vi "ALARM HIGH THRESHOLD 2.vi"(4 "State":i16=-1, 5 "Time":dbl format="%.2f", 6 "Sensor Values":dbl[](array[numeric]), 7 "Set Points":dbl[](array[numeric])=[0.0]) -> (0 "required data":T3={"Set Point names"=["Device ID"], "required number of setpoints"=1, "required number of sensors"=0, "Sensor names"=[]}, 3 "output value":dbl)   [LabVIEW 2019]
uses:
  modbusrtu/MB ID-Address.ctl
  modbusrtu/SerialParameters.ctl
  modbusrtu/MB cmd buffer.ctl
panel:
  in  "ChemTracChannels":string[](array[string])=["Acquiring", "Reserved 1", "Reserved 2", "Reserved 3", "LVAL", "CVAL", "Count Index", "Holding", "Particle Count 1 (high)", "Particle Count 1 (low)", "Particle Count 2 (high)", "Particle Count 2 (low)", "Particle Count 3 (high)", "Particle Count 3 (low)", "Particle Count 4 (high)", "Particle Count 4 (low)", "Particle Count 5 (high)", "Particle Count 5 (low)", "Particle Count 6 (high)", "Particle Count 6 (low)", "Particle Count 7 (high)", "Particle Count 7 (low)", "Particle Count 8 (high)", "Particle Count 8 (low)", "Particle Count 9 (high)", "Particle Count 9 (low)", "Total Counts (high)", "Total Counts (low)", "Alarm Output (0)", "Alarm Output (1)", "Unit Address", "Flow Rate", "Size Ranges 1 (from)", "Size Ranges 1 (to)", "Size Ranges 2 (from)", "Size Ranges 2 (to)", "Size Ranges 3 (from)", "Size Ranges 3 (to)", "Size Ranges 4 (from)", "Size Ranges 4 (to)", "Size Ranges 5 (from)", "Size Ranges 5 (to)", "Size Ranges 6 (from)", "Size Ranges 6 (to)", "Size Ranges 7 (from)", "Size Ranges 7 (to)", "Size Ranges 8 (from)", "Size Ranges 8 (to)", "Sample Frequency", "Sample Time", "CLOCK (year)", "CLOCK (month)", "CLOCK (day)", "CLOCK (hour)", "CLOCK (minute)", "CLOCK (second)", "ALARM HIGH THRESHOLD 1", "ALARM LOW THRESHOLD 1", "ALARM HIGH THRESHOLD 2", "ALARM LOW THRESHOLD 2", "ANALOG INPUT 1-1", "ANALOG INPUT 1-2", "ANALOG INPUT 1-3", "ANALOG INPUT 1-4", "ANALOG INPUT 2-1", "ANALOG INPUT 2-2", "ANALOG INPUT 2-3", "ANALOG INPUT 2-4"]
  in  "MB ID-Address in":T1={"Serial Parameter"={"Mode"=enum."RTU", "Address"=0, "Address bytes"=enum."2 bytes"}, "Start register"=0}
  # "Input Registers (Read Only)\nModbus Map: ChemTrac PC3400 Particle Counter\nAddress\tSize\tType\tDescription\t\t\t\t\t\t\t\t\t\t\t\t\t\n0\t2\tINTEGER\tAcquiring\t\t\t\t\t\t\t\t\t\t\t\t\t\n2\t2\tINTEGER\tReserved 1\t\t\t\t\t\t\t\t\t\t\t\t\t\n4\t2\tINTEGER\tReserved 2\t\t\t\t\t\t\t\t\t\t\t\t\t\n6\t2\tINTEGER\tReserved 3\t\t\t\t\t\t\t\t\t\t\t\t\t\n8\t2\tINTEGER\tLVAL\t\t\t\t\t\t\t\t\t\t\t\t\t\n10\t2\tINTEGER\tCVAL\t\t\t\t\t\t\t\t\t\t\t\t\t\n12\t2\tINTEGER\tCount Index\t\t\t\t\t\t\t\t\t\t\t\t\t\n14\t2\tINTEGER\tHolding\t\t\t\t\t\t\t\t\t\t\t\t\t\n16\t2\tINTEGER\tParticle Count 1 (high)\t\t\t\t\t\t\t\t\t\t\t\t\t\n18\t2\tINTEGER\tParticle Count 1 (low)\t\t\t\t\t\t\t\t\t\t\t\t\t\n20\t2\tINTEGER\tParticle Count 2 (high)\t\t\t\t\t\t\t\t\t\t\t\t\t\n22\t2\tINTEGER\tParticle Count 2 (low)\t\t\t\t\t\t\t\t\t\t\t\t\t\n24\t2\tINTEGER\tParticle Count 3 (high)\t\t\t\t\t\t\t\t\t\t\t\t\t\n26\t2\tINTEGER\tParticle Count 3 (low)\t\t\t\t\t\t\t\t\t\t\t\t\t\n28\t2\tINTEGER\tParticle Count 4 (high)\t\t\t\t\t\t\t\t\t\t\t\t\t\n30\t2\tINTEGER\tParticle Count 4 (low)\t\t\t\t\t\t\t\t\t\t\t\t\t\n32\t2\tINTEGER\tParticle Count 5 (high)\t\t\t\t\t\t\t\t\t\t\t\t\t\n34\t2\tINTEGER\tParticle Count 5 (low)\t\t\t\t\t\t\t\t\t\t\t\t\t\n36\t2\tINTEGER\tParticle Count 6 (high)\t\t\t\t\t\t\t\t\t\t\t\t\t\n38\t2\tINTEGER\tParticle Count 6 (low)\t\t\t\t\t\t\t\t\t\t\t\t\t\n40\t2\tINTEGER\tParticle Count 7 (high)\t\t\t\t\t\t\t\t\t\t\t\t\t\n42\t2\tINTEGER\tParticle Count 7 (low)\t\t\t\t\t\t\t\t\t\t\t\t\t\n44\t2\tINTEGER\tParticle Count 8 (high)\t\t\t\t\t\t\t\t\t\t\t\t\t\n46\t2\tINTEGER\tParticle Count 8 (low)\t\t\t\t\t\t\t\t\t\t\t\t\t\n48\t2\tINTEGER\tParticle Count 9 (high)\t\t\t\t\t\t\t\t\t\t\t\t\t\n50\t2\tINTEGER\tParticle Count 9 (low)\t\t\t\t\t\t\t\t\t\t\t\t\t\n52\t2\tINTEGER\tTotal Counts (high)\t\t\t\t\t\t\t\t\t\t\t\t\t\n54\t2\tINTEGER\tTotal Counts (low)\t\t\t\t\t\t\t\t\t\t\t\t\t\n56\t2\tINTEGER\tAlarm Output (0)\t\t\t\t\t\t\t\t\t\t\t\t\t\n58\t2\tINTEGER\tAlarm Output (1)\t\t\t\t\t\t\t\t\t\t\t\t\t\n60\t1\tINTEGER\tUnit Address\t\t\t\t\t\t\t\t\t\t\t\t\t\n62\t1\tINTEGER\tFlow Rate\t\t\t\t\t\t\t\t\t\t\t\t\t\n64\t2\tINTEGER\tSize Ranges 1 (from)\t\t\t\t\t\t\t\t\t\t\t\t\t\n66\t2\tINTEGER\tSize Ranges 1 (to)\t\t\t\t\t\t\t\t\t\t\t\t\t\n68\t2\tINTEGER\tSize Ranges 2 (from)\t\t\t\t\t\t\t\t\t\t\t\t\t\n70\t2\tINTEGER\tSize Ranges 2 (to)\t\t\t\t\t\t\t\t\t\t\t\t\t\n72\t2\tINTEGER\tSize Ranges 3 (from)\t\t\t\t\t\t\t\t\t\t\t\t\t\n74\t2\tINTEGER\tSize Ranges 3 (to)\t\t\t\t\t\t\t\t\t\t\t\t\t\n76\t2\tINTEGER\tSize Ranges 4 (from)\t\t\t\t\t\t\t\t\t\t\t\t\t\n78\t2\tINTEGER\tSize Ranges 4 (to)\t\t\t\t\t\t\t\t\t\t\t\t\t\n80\t2\tINTEGER\tSize Ranges 5 (from)\t\t\t\t\t\t\t\t\t\t\t\t\t\n82\t2\tINTEGER\tSize Ranges 5 (to)\t\t\t\t\t\t\t\t\t\t\t\t\t\n84\t2\tINTEGER\tSize Ranges 6 (from)\t\t\t\t\t\t\t\t\t\t\t\t\t\n86\t2\tINTEGER\tSize Ranges 6 (to)\t\t\t\t\t\t\t\t\t\t\t\t\t\n88\t2\tINTEGER\tSize Ranges 7 (from)\t\t\t\t\t\t\t\t\t\t\t\t\t\n90\t2\tINTEGER\tSize Ranges 7 (to)\t\t\t\t\t\t\t\t\t\t\t\t\t\n92\t2\tINTEGER\tSize Ranges 8 (from)\t\t\t\t\t\t\t\t\t\t\t\t\t\n94\t2\tINTEGER\tSize Ranges 8 (to)\t\t\t\t\t\t\t\t\t\t\t\t\t\n96\t2\tINTEGER\tSample Frequency\t\t\t\t\t\t\t\t\t\t\t\t\t\n98\t2\tINTEGER\tSample Time\t\t\t\t\t\t\t\t\t\t\t\t\t\n100\t2\tINTEGER\tCLOCK (year)\t\t\t\t\t\t\t\t\t\t\t\t\t\n102\t2\tINTEGER\tCLOCK (month)\t\t\t\t\t\t\t\t\t\t\t\t\t\n104\t2\tINTEGER\tCLOCK (day)\t\t\t\t\t\t\t\t\t\t\t\t\t\n106\t2\tINTEGER\tCLOCK (hour)\t\t\t\t\t\t\t\t\t\t\t\t\t\n108\t2\tINTEGER\tCLOCK (minute)\t\t\t\t\t\t\t\t\t\t\t\t\t\n110\t2\tINTEGER\tCLOCK (second)\t\t\t\t\t\t\t\t\t\t\t\t\t\n112\t2\tINTEGER\tALARM HIGH THRESHOLD 1\t\t\t\t\t\t\t\t\t\t\t\t\t\n114\t2\tINTEGER\tALARM LOW THRESHOLD 1\t\t\t\t\t\t\t\t\t\t\t\t\t\n116\t2\tINTEGER\tALARM HIGH THRESHOLD 2\t\t\t\t\t\t\t\t\t\t\t\t\t\n118\t2\tINTEGER\tALARM LOW THRESHOLD 2\t\t\t\t\t\t\t\t\t\t\t\t\t\n120\t2\tINTEGER\tANALOG INPUT 1-1\t\t\t\t\t\t\t\t\t\t\t\t\t\n122\t2\tINTEGER\tANALOG INPUT 1-2\t\t\t\t\t\t\t\t\t\t\t\t\t\n124\t2\tINTEGER\tANALOG INPUT 1-3\t\t\t\t\t\t\t\t\t\t\t\t\t\n126\t2\tINTEGER\tANALOG INPUT 1-4\t\t\t\t\t\t\t\t\t\t\t\t\t\n128\t2\tINTEGER\tANALOG INPUT 2-1\t\t\t\t\t\t\t\t\t\t\t\t\t\n130\t2\tINTEGER\tANALOG INPUT 2-2\t\t\t\t\t\t\t\t\t\t\t\t\t\n132\t2\tINTEGER\tANALOG INPUT 2-3\t\t\t\t\t\t\t\t\t\t\t\t\t\n134\t2\tINTEGER\tANALOG INPUT 2-4"
  # "Enter the correct information for this control code in the required data structure below. Then make the current value default by right clicking on the border of the data structure. Select \"data operations\" and then select \"make current value default\". These values will be displayed by process controller."
  # "HydroACT has even parity by default."
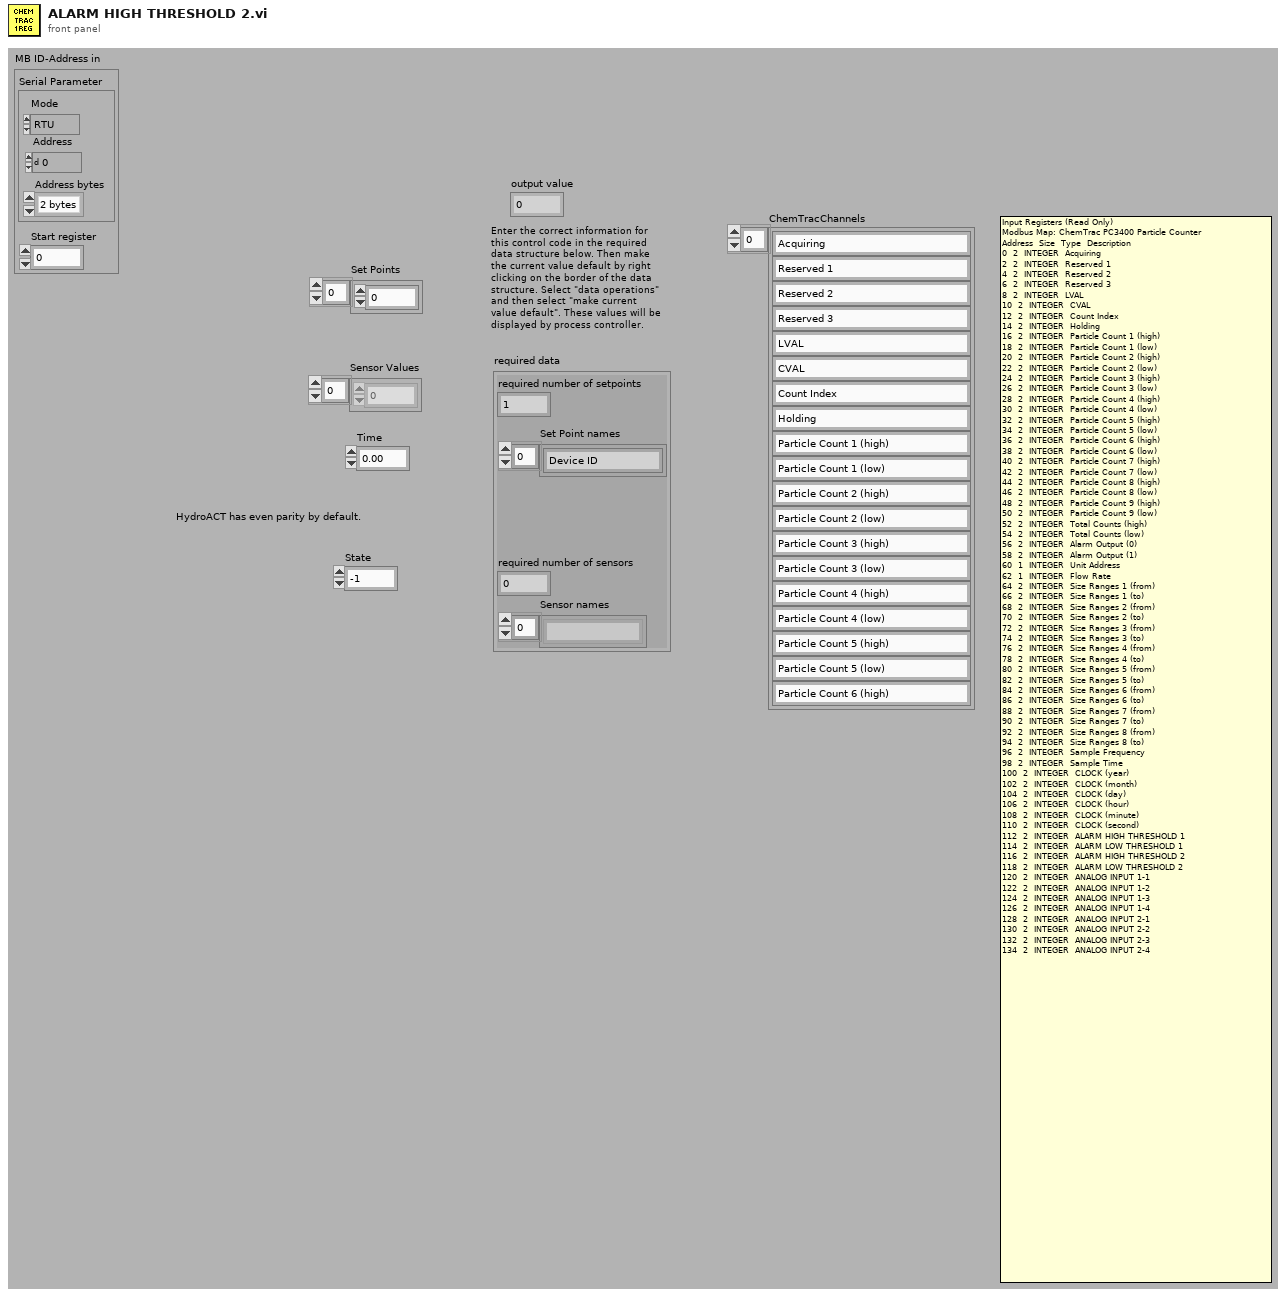
[diagram p1: front panel]
types:
  T1 = typedef "MB ID-Address.ctl" = cluster{"Serial Parameter":T2, "Start register":u16}
  T2 = typedef "SerialParameters.ctl" = cluster{"Mode":enum16{"RTU", "ASCII"}, "Address":u16, "Address bytes":enum16{"1 byte", "2 bytes"}}
  T3 = cluster{"Set Point names":string[], "required number of setpoints":u8, "required number of sensors":u8, "Sensor names":string[]}
  T4 = typedef "MB cmd buffer.ctl" = enum16{"ProCoDA", "MB succeed", "MB error", "MB Next Task", "ProCoDA read 1", "Commands pending"}
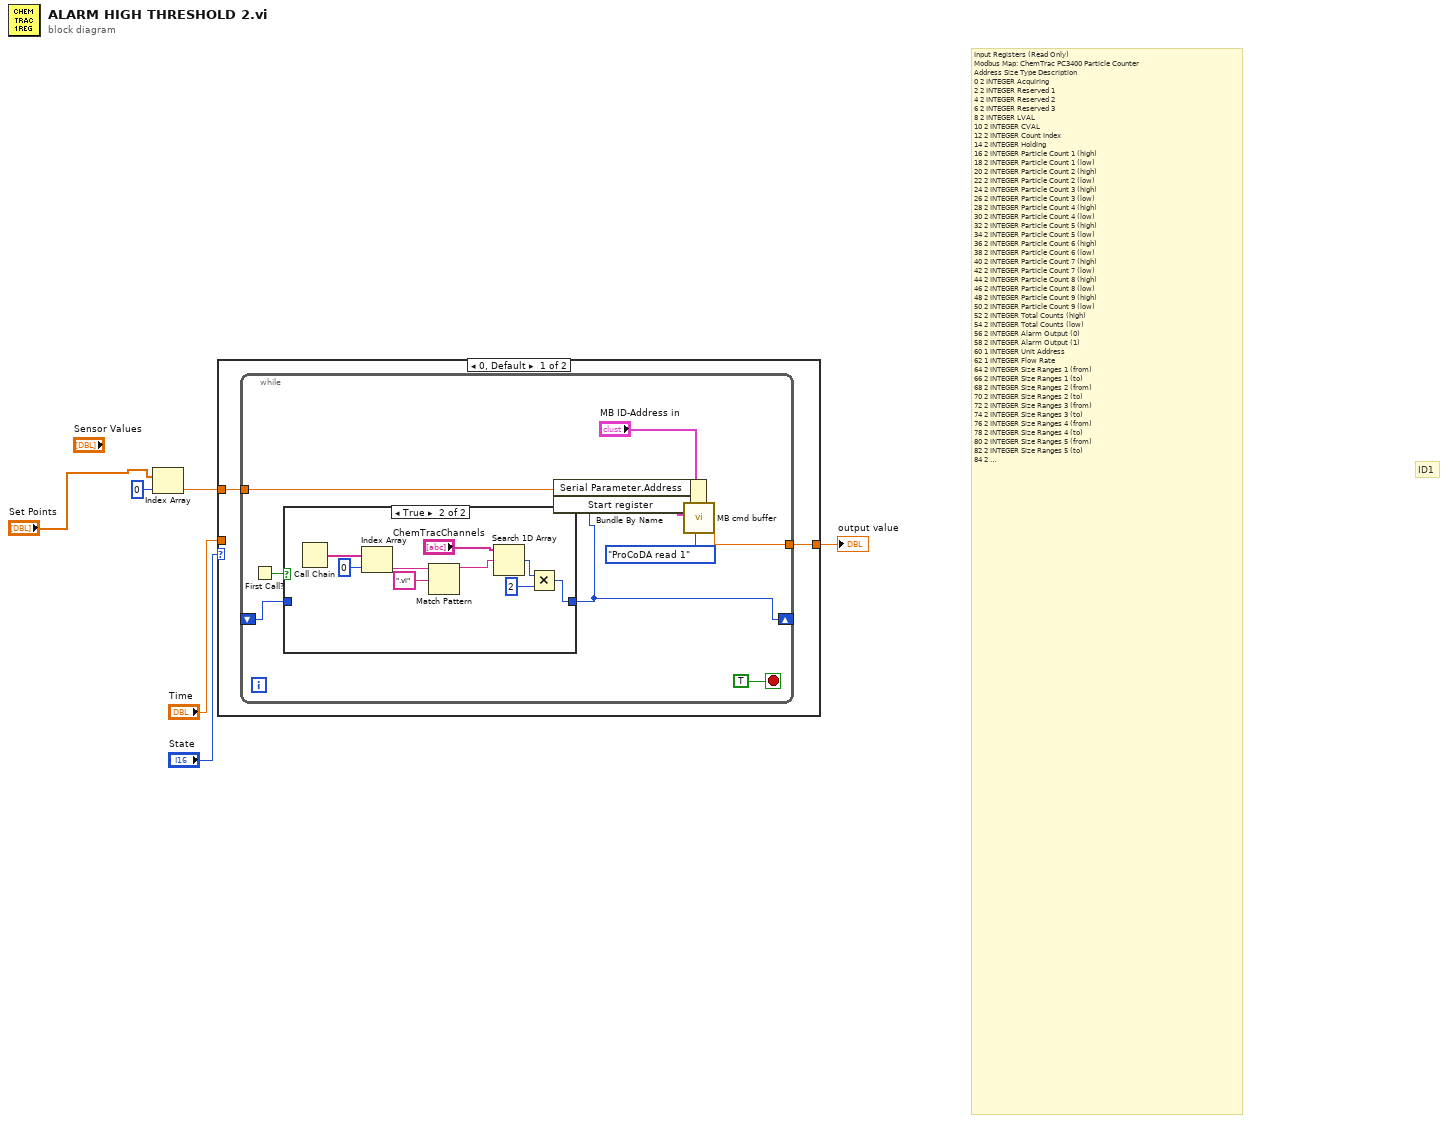
[diagram p0: block diagram]
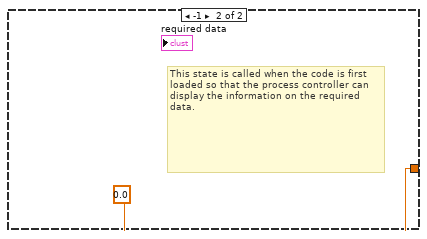
[diagram p3: hidden frame]
diagram:
  # "Input Registers (Read Only)\nModbus Map: ChemTrac PC3400 Particle Counter\nAddress\tSize\tType\tDescription\t\t\t\t\t\t\t\t\t\t\t\t\t\n0\t2\tINTEGER\tAcquiring\t\t\t\t\t\t\t\t\t\t\t\t\t\n2\t2\tINTEGER\tReserved 1\t\t\t\t\t\t\t\t\t\t\t\t\t\n4\t2\tINTEGER\tReserved 2\t\t\t\t\t\t\t\t\t\t\t\t\t\n6\t2\tINTEGER\tReserved 3\t\t\t\t\t\t\t\t\t\t\t\t\t\n8\t2\tINTEGER\tLVAL\t\t\t\t\t\t\t\t\t\t\t\t\t\n10\t2\tINTEGER\tCVAL\t\t\t\t\t\t\t\t\t\t\t\t\t\n12\t2\tINTEGER\tCount Index\t\t\t\t\t\t\t\t\t\t\t\t\t\n14\t2\tINTEGER\tHolding\t\t\t\t\t\t\t\t\t\t\t\t\t\n16\t2\tINTEGER\tParticle Count 1 (high)\t\t\t\t\t\t\t\t\t\t\t\t\t\n18\t2\tINTEGER\tParticle Count 1 (low)\t\t\t\t\t\t\t\t\t\t\t\t\t\n20\t2\tINTEGER\tParticle Count 2 (high)\t\t\t\t\t\t\t\t\t\t\t\t\t\n22\t2\tINTEGER\tParticle Count 2 (low)\t\t\t\t\t\t\t\t\t\t\t\t\t\n24\t2\tINTEGER\tParticle Count 3 (high)\t\t\t\t\t\t\t\t\t\t\t\t\t\n26\t2\tINTEGER\tParticle Count 3 (low)\t\t\t\t\t\t\t\t\t\t\t\t\t\n28\t2\tINTEGER\tParticle Count 4 (high)\t\t\t\t\t\t\t\t\t\t\t\t\t\n30\t2\tINTEGER\tParticle Count 4 (low)\t\t\t\t\t\t\t\t\t\t\t\t\t\n32\t2\tINTEGER\tParticle Count 5 (high)\t\t\t\t\t\t\t\t\t\t\t\t\t\n34\t2\tINTEGER\tParticle Count 5 (low)\t\t\t\t\t\t\t\t\t\t\t\t\t\n36\t2\tINTEGER\tParticle Count 6 (high)\t\t\t\t\t\t\t\t\t\t\t\t\t\n38\t2\tINTEGER\tParticle Count 6 (low)\t\t\t\t\t\t\t\t\t\t\t\t\t\n40\t2\tINTEGER\tParticle Count 7 (high)\t\t\t\t\t\t\t\t\t\t\t\t\t\n42\t2\tINTEGER\tParticle Count 7 (low)\t\t\t\t\t\t\t\t\t\t\t\t\t\n44\t2\tINTEGER\tParticle Count 8 (high)\t\t\t\t\t\t\t\t\t\t\t\t\t\n46\t2\tINTEGER\tParticle Count 8 (low)\t\t\t\t\t\t\t\t\t\t\t\t\t\n48\t2\tINTEGER\tParticle Count 9 (high)\t\t\t\t\t\t\t\t\t\t\t\t\t\n50\t2\tINTEGER\tParticle Count 9 (low)\t\t\t\t\t\t\t\t\t\t\t\t\t\n52\t2\tINTEGER\tTotal Counts (high)\t\t\t\t\t\t\t\t\t\t\t\t\t\n54\t2\tINTEGER\tTotal Counts (low)\t\t\t\t\t\t\t\t\t\t\t\t\t\n56\t2\tINTEGER\tAlarm Output (0)\t\t\t\t\t\t\t\t\t\t\t\t\t\n58\t2\tINTEGER\tAlarm Output (1)\t\t\t\t\t\t\t\t\t\t\t\t\t\n60\t1\tINTEGER\tUnit Address\t\t\t\t\t\t\t\t\t\t\t\t\t\n62\t1\tINTEGER\tFlow Rate\t\t\t\t\t\t\t\t\t\t\t\t\t\n64\t2\tINTEGER\tSize Ranges 1 (from)\t\t\t\t\t\t\t\t\t\t\t\t\t\n66\t2\tINTEGER\tSize Ranges 1 (to)\t\t\t\t\t\t\t\t\t\t\t\t\t\n68\t2\tINTEGER\tSize Ranges 2 (from)\t\t\t\t\t\t\t\t\t\t\t\t\t\n70\t2\tINTEGER\tSize Ranges 2 (to)\t\t\t\t\t\t\t\t\t\t\t\t\t\n72\t2\tINTEGER\tSize Ranges 3 (from)\t\t\t\t\t\t\t\t\t\t\t\t\t\n74\t2\tINTEGER\tSize Ranges 3 (to)\t\t\t\t\t\t\t\t\t\t\t\t\t\n76\t2\tINTEGER\tSize Ranges 4 (from)\t\t\t\t\t\t\t\t\t\t\t\t\t\n78\t2\tINTEGER\tSize Ranges 4 (to)\t\t\t\t\t\t\t\t\t\t\t\t\t\n80\t2\tINTEGER\tSize Ranges 5 (from)\t\t\t\t\t\t\t\t\t\t\t\t\t\n82\t2\tINTEGER\tSize Ranges 5 (to)\t\t\t\t\t\t\t\t\t\t\t\t\t\n84\t2\tINTEGER\tSize Ranges 6 (from)\t\t\t\t\t\t\t\t\t\t\t\t\t\n86\t2\tINTEGER\tSize Ranges 6 (to)\t\t\t\t\t\t\t\t\t\t\t\t\t\n88\t2\tINTEGER\tSize Ranges 7 (from)\t\t\t\t\t\t\t\t\t\t\t\t\t\n90\t2\tINTEGER\tSize Ranges 7 (to)\t\t\t\t\t\t\t\t\t\t\t\t\t\n92\t2\tINTEGER\tSize Ranges 8 (from)\t\t\t\t\t\t\t\t\t\t\t\t\t\n94\t2\tINTEGER\tSize Ranges 8 (to)\t\t\t\t\t\t\t\t\t\t\t\t\t\n96\t2\tINTEGER\tSample Frequency\t\t\t\t\t\t\t\t\t\t\t\t\t\n98\t2\tINTEGER\tSample Time\t\t\t\t\t\t\t\t\t\t\t\t\t\n100\t2\tINTEGER\tCLOCK (year)\t\t\t\t\t\t\t\t\t\t\t\t\t\n102\t2\tINTEGER\tCLOCK (month)\t\t\t\t\t\t\t\t\t\t\t\t\t\n104\t2\tINTEGER\tCLOCK (day)\t\t\t\t\t\t\t\t\t\t\t\t\t\n106\t2\tINTEGER\tCLOCK (hour)\t\t\t\t\t\t\t\t\t\t\t\t\t\n108\t2\tINTEGER\tCLOCK (minute)\t\t\t\t\t\t\t\t\t\t\t\t\t\n110\t2\tINTEGER\tCLOCK (second)\t\t\t\t\t\t\t\t\t\t\t\t\t\n112\t2\tINTEGER\tALARM HIGH THRESHOLD 1\t\t\t\t\t\t\t\t\t\t\t\t\t\n114\t2\tINTEGER\tALARM LOW THRESHOLD 1\t\t\t\t\t\t\t\t\t\t\t\t\t\n116\t2\tINTEGER\tALARM HIGH THRESHOLD 2\t\t\t\t\t\t\t\t\t\t\t\t\t\n118\t2\tINTEGER\tALARM LOW THRESHOLD 2\t\t\t\t\t\t\t\t\t\t\t\t\t\n120\t2\tINTEGER\tANALOG INPUT 1-1\t\t\t\t\t\t\t\t\t\t\t\t\t\n122\t2\tINTEGER\tANALOG INPUT 1-2\t\t\t\t\t\t\t\t\t\t\t\t\t\n124\t2\tINTEGER\tANALOG INPUT 1-3\t\t\t\t\t\t\t\t\t\t\t\t\t\n126\t2\tINTEGER\tANALOG INPUT 1-4\t\t\t\t\t\t\t\t\t\t\t\t\t\n128\t2\tINTEGER\tANALOG INPUT 2-1\t\t\t\t\t\t\t\t\t\t\t\t\t\n130\t2\tINTEGER\tANALOG INPUT 2-2\t\t\t\t\t\t\t\t\t\t\t\t\t\n132\t2\tINTEGER\tANALOG INPUT 2-3\t\t\t\t\t\t\t\t\t\t\t\t\t\n134\t2\tINTEGER\tANALOG INPUT 2-4"
  # "ID1"
  n1 = Index Array(array="Set Points", index=0) -> (element=w2:dbl)
  n2 = case shown="0, Default" "State" {
    tunnel: [w8 0.0 ("fraction on")] -> w5
    tunnel: "Time" -> [_ _]
    tunnel: w2 -> [w7 _]
    frame 0, Default {
      n3 = while {
        tunnel: [w16] -> w8
        tunnel: w7 -> [w13]
        shift-right: [w11] -> _
        shift-left: _ -> [w10]
        stop <- TRUE stop-if-true
        n4 = First Call?() -> (First Call?: T/F=w12:bool)
        n5 = case shown="True" w12 {
          tunnel: [w18 w20] -> w11
          tunnel: w10 -> [w18 _]
          frame False {
          }
          frame True {
            n6 = Call Chain() -> (call chain=w26:string[])
            n7 = Index Array(array=w26, index=0) -> (element=w27:string)
            n8 = Match Pattern(string=w27, regular expression=".vi") -> (before substring=w23:string)  [unwired: 1 in, 3 out]
            n9 = Search 1D Array(1D array="ChemTracChannels", element=w23) -> (index of element=w22:i32)  [unwired: 1 in]
            n10 = Multiply(x=w22, y=2) -> (x*y=w20:i32)
          }
        }
        n11 = Bundle By Name(cluster="MB ID-Address in", "Serial Parameter.Address"=w13, "Start register"=w11) -> (w14:T1)
        n12 = call "MB cmd buffer.vi"("MB cmd buffer"=MB_cmd_buffer."ProCoDA read 1", "MB ID-Address in"=w14) -> ("output value"=w16:dbl)  [unwired: 3 in, 6 out]
      }
    }
    frame -1 {
      # "This state is called when the code is first loaded so that the process controller can display the information on the required data."
    }
  }
  "output value" <- w5
